vi "Find Resource by Type.vi"   [LabVIEW 2017]
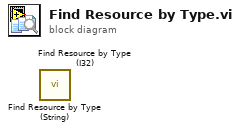
[diagram p0: block diagram]
diagram:
  n1 = call "Find Resource by Type (String).vi"() -> ()  [unwired: 9 in, 3 out]
  n2 = call "Find Resource by Type (I32).vi"() -> ()  [unwired: 9 in, 3 out]
